vi "clean_both_channels.vi"(0 "Detector in":refnum<class "Detector.lvclass">, 1 "I channel seq IN in":cluster{"BG":sgl[], "Ie":sgl[], "I0":sgl[]}[](array[cluster]), 3 "II channel seq IN in":cluster{"BG":sgl[], "Ie":sgl[], "I0":sgl[]}[](array[cluster]), 5 "I channel":sgl[][](array[numeric]), 9 "II channel":sgl[][](array[numeric]), 11 "error in (no error)":errorcluster, 12 "All?":bool, 14 "# of scan":i32) -> (4 "Detector out":refnum<class "Detector.lvclass">, 6 "I channel seq IN out":cluster{"BG":sgl[], "Ie":sgl[], "I0":sgl[]}[](array[cluster]), 8 "BG indexes":i32[](array[numeric]), 10 "II channel seq IN out":cluster{"BG":sgl[], "Ie":sgl[], "I0":sgl[]}[](array[cluster]), 15 "error out":errorcluster)   [LabVIEW 2020, in "Detector.lvclass"]
uses:
  Detector.lvclass
  Detector.lvclass/Detector.ctl
  Read SC sum values ref.vi
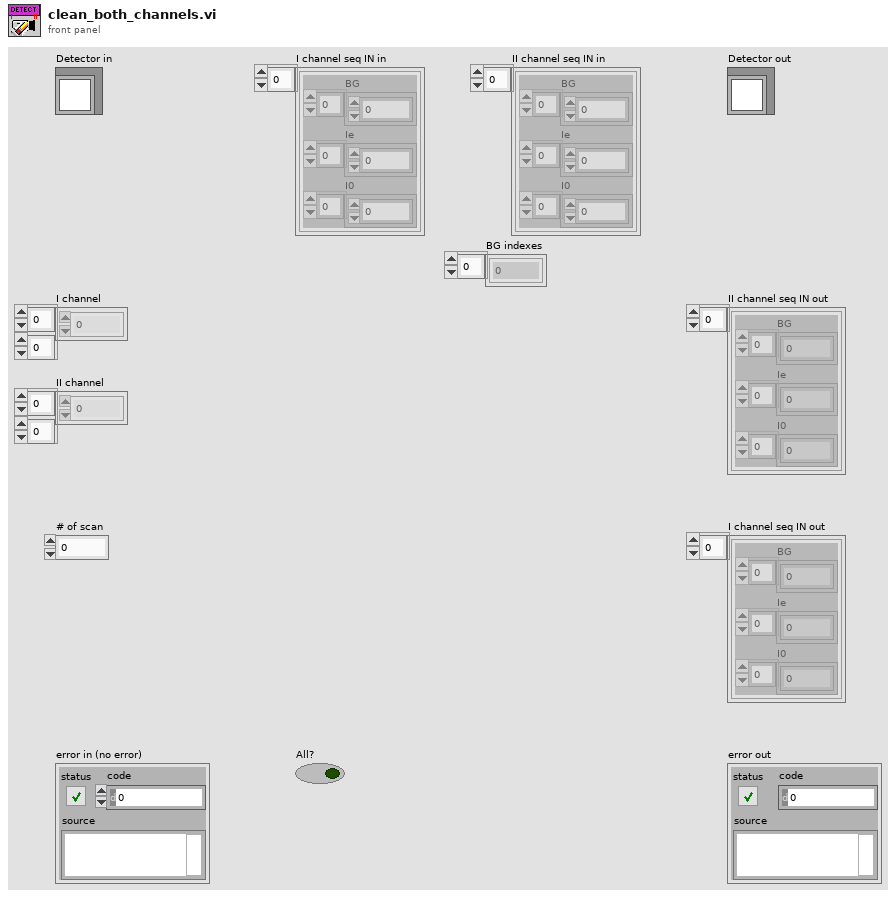
[diagram p1: front panel]
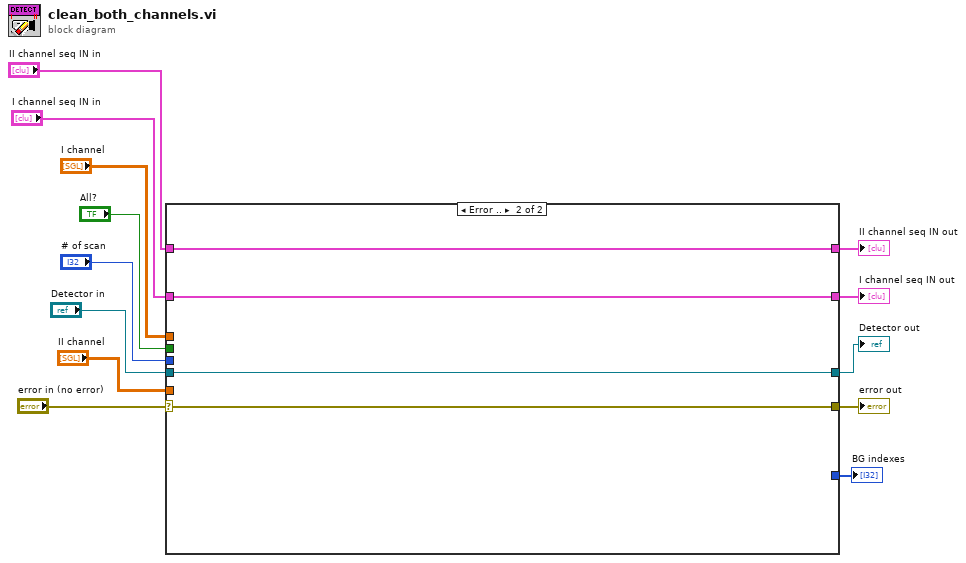
[diagram p0: block diagram]
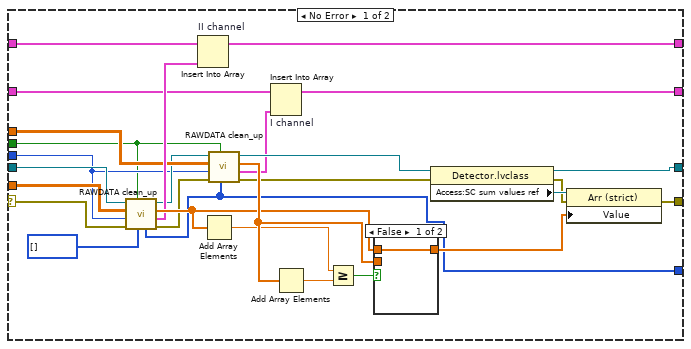
[diagram p2: hidden frame]
diagram:
  n1 = case shown="Error .." "error in (no error)" {
    selector: "error in (no error)" -> [w18 w47]
    tunnel: [w41 w47] -> w13
    tunnel: [w39 w45] -> w12
    tunnel: [w38 w46] -> w11
    tunnel: "I channel" -> [w30 _]
    tunnel: "II channel" -> [w29 _]
    tunnel: "Detector in" -> [w21 w44]
    tunnel: "I channel seq IN in" -> [w20 w46]
    tunnel: "II channel seq IN in" -> [w19 w45]
    tunnel: [w17 w44] -> w4
    tunnel: "# of scan" -> [w16 _]
    tunnel: "All?" -> [w15 _]
    tunnel: [w14 _] -> w1
    frame No Error {
      n2 = call "RAWDATA clean_up.vi"("BG index IN"=i32[] [], "All?"=w15, "error in (no error)"=w18, "# of scan"=w16, "channel"=w29, "Detector in"=w21) -> ("error out"=w27:errorcluster, "channel seq"=w32:cluster{"BG":i32[], "Ie":i32[], "I0":i32[]}[], "SC values"=w36:sgl[], "Detector out"=w28:refnum<class "Detector.lvclass">, "BG indexes"=w14:i32[])  [unwired: 1 in]
      n3 = Insert Into Array "II channel"(array=w19, new element=w32) -> (w39:cluster{"BG":sgl[], "Ie":sgl[], "I0":sgl[]}[])  [unwired: 1 in]
      n4 = Add Array Elements(numeric array=w36) -> (sum=w24:sgl)
      n5 = call "RAWDATA clean_up.vi"("BG index IN"=w14, "All?"=w15, "error in (no error)"=w27, "# of scan"=w16, "channel"=w30, "Detector in"=w28) -> ("error out"=w34:errorcluster, "channel seq"=w31:cluster{"BG":i32[], "Ie":i32[], "I0":i32[]}[], "SC values"=w40:sgl[], "Detector out"=w33:refnum<class "Detector.lvclass">)  [unwired: 1 in, 1 out]
      n6 = Insert Into Array "I channel"(array=w20, new element=w31) -> (w38:cluster{"BG":sgl[], "Ie":sgl[], "I0":sgl[]}[])  [unwired: 1 in]
      n7 = Add Array Elements(numeric array=w40) -> (sum=w25:sgl)
      n8 = Greater Or Equal?(x=w24, y=w25) -> (x >= y?=w26:bool)
      n9 = case shown="False" w26 {
        tunnel: w36 -> [w42 _]
        tunnel: [w42 w43] -> w35
        tunnel: w40 -> [_ w43]
        frame False {
        }
        frame True {
        }
      }
      n10 = property class="Detector.lvclass"(reference=w33, error in=w34) -> (reference out=w17:refnum<class "Detector.lvclass">, error out=w22:errorcluster, "Access:SC sum values ref"=w23:refnum<vi>)
      n11 = property class="Arr (strict)"(reference=w23, error in=w22, "Value"=w35) -> (error out=w41:errorcluster)  [unwired: 1 out]
    }
    frame Error {
    }
  }
  "error out" <- w13
  "II channel seq IN out" <- w12
  "I channel seq IN out" <- w11
  "Detector out" <- w4
  "BG indexes" <- w1
